vi "Launch Async.vi"(7 "Wait to Start":bool, 8 "error in (no error)":errorcluster, 10 "Caller Queue":refnum<class "Priority Message Queue.lvclass">, 11 "Actor in":refnum<class "Actor.lvclass">) -> (0 "error out":errorcluster, 2 "Actor API":refnum<class "Actor API.lvclass">)   [LabVIEW 2020, in "Artifex.lvlib" / "Actor.lvclass"]
doc: "Equivalent of Actor.vi"
uses:
  Actor.lvclass
  Actor Async.vi
  Actor Proxy/Actor API.lvclass
  Priority Message Queue/Priority Message Queue.lvclass
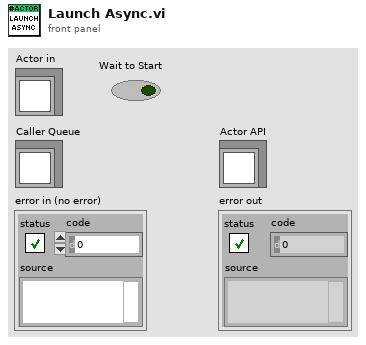
[diagram p1: front panel]
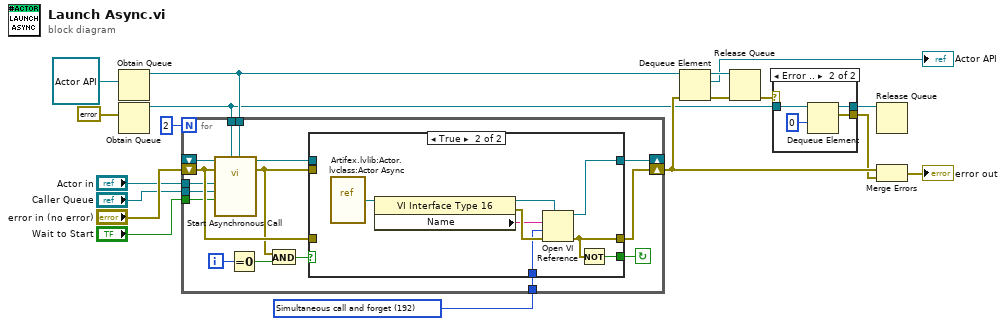
[diagram p0: block diagram]
diagram:
  w15 = 192 items=["Record modifications"=1, "Open templates for editing"=2, "Prompt user to save"=4, "Prepare for reentrant run"=8, "Prompt to find missing subVIs"=16, "Hide loading dialog box"=32, "Enable simultaneous calls"=64, "Prepare to call and forget"=128, "Simultaneous call and forget"=192, "Prepare to call and collect"=256, "Simultaneous call and collect"=320]
  n1 = Obtain Queue(element data type=refnum<class "Actor API.lvclass"> refnum ("Artifex.lvlib:Actor API.lvclass")) -> (queue out=w9:refnum<queue>)  [unwired: 4 in, 2 out]
  n2 = Obtain Queue(element data type=errorcluster {"status"=FALSE, "code"=0, "source"=""} ("error constant")) -> (queue out=w4:refnum<queue>)  [unwired: 4 in, 2 out]
  n3 = for {
    N: 2 -> [_]
    tunnel: w15 -> [w30]
    shift-right: [w29] -> _
    shift-left: _ -> [w28]
    shift-right: [w26] -> w8
    shift-left: "error in (no error)" -> [w25]
    tunnel: w4 -> [w23]
    tunnel: "Actor in" -> [w22]
    tunnel: w9 -> [w21]
    tunnel: "Caller Queue" -> [w20]
    tunnel: "Wait to Start" -> [w19]
    i -> [w34]
    stop <- w27 continue-if-true
    n4 = call-by-ref "Start Asynchronous Call"(reference=w28, error in=w25, "API Q"=w21, "Error Q"=w23, "Wait Core"=w19, "Caller Queue"=w20, "Actor in"=w22) -> (reference out=w31:refnum<vi>, error out=w24:errorcluster)  [unwired: 7 in]
    n5 = Equal To 0?(x=w34) -> (x = 0?=w33:bool)
    n6 = And(x=w24, y=w33) -> (x .and. y?=w32:bool)
    n7 = case shown="True" w32 {
      tunnel: w31 -> [w36 _]
      tunnel: w30 -> [_ w41]
      tunnel: [w36 w39] -> w29
      tunnel: [_ w38] -> w27
      tunnel: [w35 w37] -> w26
      tunnel: w25 -> [w35 _]
      tunnel: w24 -> [_ _]
      frame False {
      }
      frame True {
        n8 = vi-ref "Artifex.lvlib:Actor.lvclass:Actor Async.vi"() -> (w43:refnum<vi>)
        n9 = property class="VI Interface Type 16"(reference=w43) -> (reference out=w40:refnum<vi>, error out=w44:errorcluster, "Name"=w42:string)  [unwired: 1 in]
        n10 = Open VI Reference(type specifier VI Refnum (for type only)=w40, vi path=w42, options=w41, error in (no error)=w44) -> (vi reference=w39:refnum<vi>, error out=w37:errorcluster)  [unwired: 2 in]
        n11 = Not(x=w37) -> (.not. x?=w38:bool)
      }
    }
  }
  n12 = Dequeue Element(queue=w9, error in (no error)=w8) -> (queue out=w7:refnum<queue>, element=→"Actor API":refnum<class "Actor API.lvclass">, error out=w6:errorcluster)  [unwired: 1 in, 1 out]
  n13 = Release Queue(queue=w7, error in (no error)=w6) -> (error out=w5:errorcluster)  [unwired: 1 in, 2 out]
  n14 = case shown="Error .." w5 {
    selector: w5 -> [w46 _]
    tunnel: w4 -> [w45 w50]
    tunnel: [w46 w48] -> w2
    tunnel: [w45 w47] -> w1
    frame No Error {
    }
    frame Error {
      n15 = Dequeue Element(queue=w50, timeout in ms (-1)=0) -> (queue out=w47:refnum<queue>, element=w48:errorcluster)  [unwired: 1 in, 2 out]
    }
  }
  n16 = Release Queue(queue=w1) -> ()  [unwired: 2 in, 3 out]
  n17 = Merge Errors(w8, w2) -> (→"error out":errorcluster)
